vi "Write SelTileCode.vi"(8 "error in (no error)":errorcluster, 10 "SelTileCode":string, 11 "Menu in":refnum<class "Menu.lvclass">) -> (0 "error out":errorcluster, 3 "Menu out":refnum<class "Menu.lvclass">)   [LabVIEW 2019, in "RT_Game.lvlib" / "Menu.lvclass"]
uses:
  Menu.lvclass
  Menu.lvclass/Menu.ctl
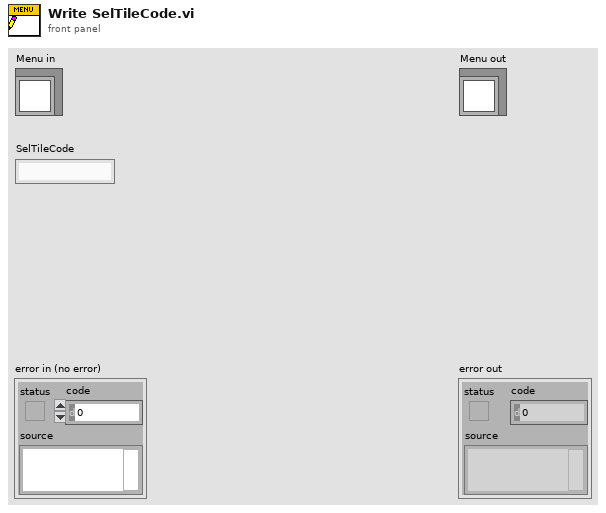
[diagram p1: front panel]
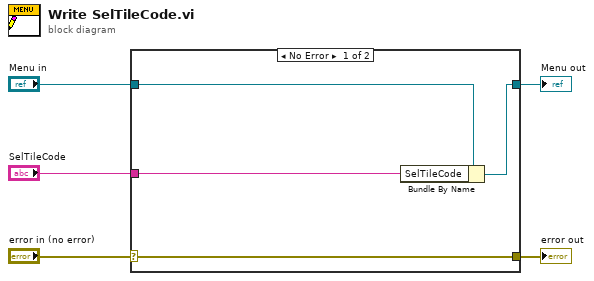
[diagram p0: block diagram]
diagram:
  n1 = case shown="No Error" "error in (no error)" {
    selector: "error in (no error)" -> [w9 w10]
    tunnel: [w9 w10] -> w4
    tunnel: [w7 w11] -> w2
    tunnel: "Menu in" -> [w8 w11]
    tunnel: "SelTileCode" -> [w6 _]
    frame No Error {
      n2 = Bundle By Name(cluster=w8, "SelTileCode"=w6) -> (w7:refnum<class "Menu.lvclass">)
    }
    frame Error {
    }
  }
  "error out" <- w4
  "Menu out" <- w2
